vi "_CSMObj-Remove Internal Registry Rule.vi"(8 "Error In":errorcluster caption="Error in (no error)", 10 "Rule":string, 11 "CSMQ In":T1={"info"={"Module Name"="", "Requested Name"="", "Group Name"="", "Mode"=enum."Stand Alone", "Allowed Messages"=[]}, "Refs"={"WatchDogQ"=refnum, "CSMDataDVR"=refnum, "Queue"={"HPriorityQ"=refnum, "LowPriorityQ"=refnum}, "GroupDataDVR"=refnum, "TagMap"=refnum, "ExitEvent"=refnum, "NewStateEvent"=refnum, "StatusEvent"=refnum, "InterruptEvent"=refnum}}) -> (0 "Error Out":errorcluster, 3 "CSMQ Out":T1={"info"={"Module Name"="", "Requested Name"="", "Group Name"="", "Mode"=enum."Stand Alone", "Allowed Messages"=[]}, "Refs"={"WatchDogQ"=refnum, "CSMDataDVR"=refnum, "Queue"={"HPriorityQ"=refnum, "LowPriorityQ"=refnum}, "GroupDataDVR"=refnum, "TagMap"=refnum, "ExitEvent"=refnum, "NewStateEvent"=refnum, "StatusEvent"=refnum, "InterruptEvent"=refnum}})   [LabVIEW 2017, in "Communicable State Machine.lvlib"]
uses:
  Communicable State Machine.lvlib
  _CSMObj.ctl
  _CSMObj-Info.ctl
  Typedef/_CSM_MODE.ctl
  _CSMObj-Refs.ctl
  _CSMObj-Data.ctl
  Priority Queue/Priority Queue.ctl
  Typedef/_Cross CSM State Data.ctl
  Typedef/_CSM_MSG_TYPE.ctl
  Typedef/_Cross CSM State Response.ctl
  Typedef/_CSM_Response Source Message.ctl
  Priority Queue/def-Data(LowPRI-Q).ctl
  _CSMObj-ModeData.ctl
  Typedef/_CSM Status Change Event Data.ctl
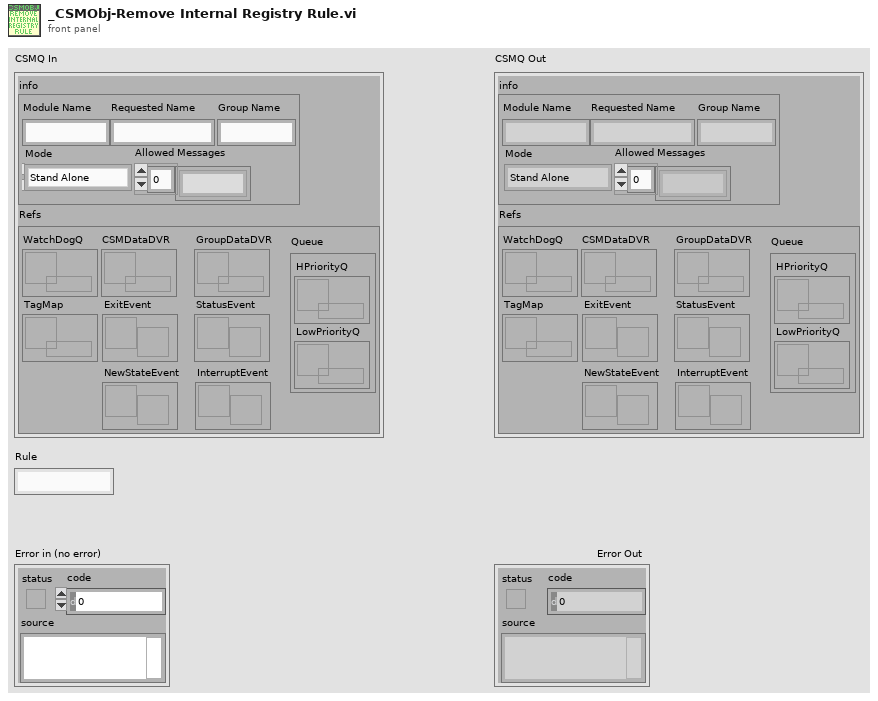
[diagram p1: front panel]
types:
  T1 = typedef "Communicable State Machine.lvlib/_CSMObj.ctl" = cluster{"info":T2, "Refs":T4}
  T2 = typedef "Communicable State Machine.lvlib/_CSMObj-Info.ctl" = cluster{"Module Name":string, "Requested Name":string, "Group Name":string, "Mode":T3, "Allowed Messages":string[]}
  T3 = typedef "Communicable State Machine.lvlib/_CSM_MODE.ctl" = enum16{"Not Exist", "Stand Alone", "CSM", "Worker", "Worker Agent", "Chain Node", "Chain"}
  T4 = typedef "Communicable State Machine.lvlib/_CSMObj-Refs.ctl" = cluster{"WatchDogQ":refnum<queue>, "CSMDataDVR":refnum<data-value>, "Queue":T5, "GroupDataDVR":refnum<data-value>, "TagMap":refnum<data-value>, "ExitEvent":refnum<user-event>, "NewStateEvent":refnum<user-event>, "StatusEvent":refnum<user-event>, "InterruptEvent":refnum<user-event>}
  T5 = typedef "Communicable State Machine.lvlib/Priority Queue.ctl" = cluster{"HPriorityQ":refnum<queue>, "LowPriorityQ":refnum<queue>}
  T6 = typedef "Communicable State Machine.lvlib/_CSMObj-Data.ctl" = cluster{"RemoteMessge?":bool, "error":errorcluster, "Return State":string, "Initialized":enum16{"Initializing", "Ready", "Exiting"}, "InternalRegistryRules":string[]}
  T7 = typedef "Communicable State Machine.lvlib/_CSMObj-ModeData.ctl" = cluster{"CSMDataDVR":refnum<data-value>[], "PriorityQueues":T5[], "Messages of Chain Nodes":cluster{"Module Name":string, "Allowed Messages":string[]}[], "Chain Message Mapping Map":variant, "SharedRegistryRules":string[]}
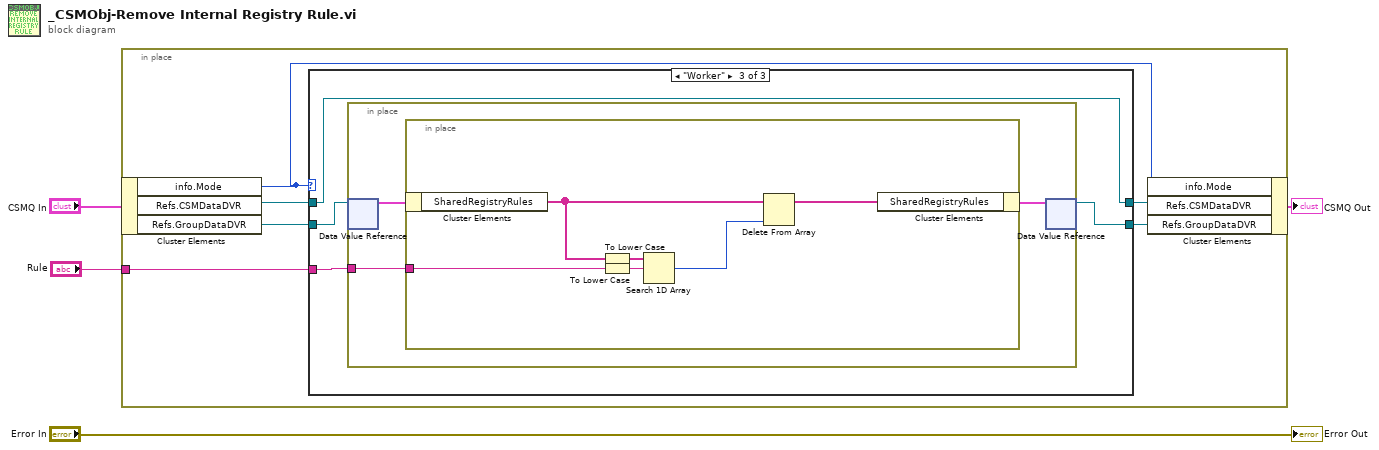
[diagram p0: block diagram]
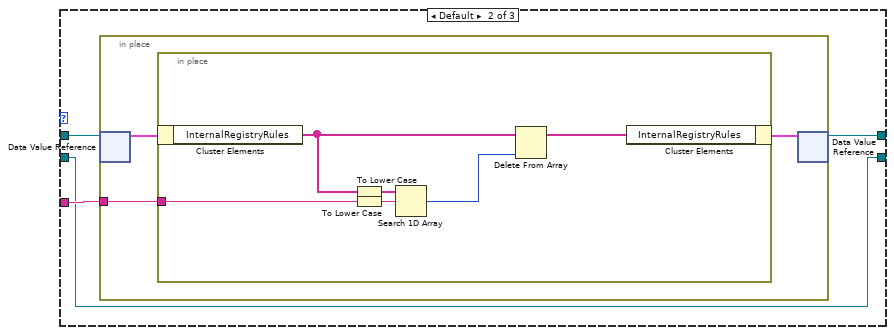
[diagram p3: hidden frame]
diagram:
  n1 = in-place "In Place Element Structure" {
    in-place-border: "Rule" -> [w8]
    n2 = in-place-cluster #1("CSMQ In") -> ("info.Mode"=w7:T3, "Refs.CSMDataDVR"=w10:refnum<data-value>, "Refs.GroupDataDVR"=w6:refnum<data-value>)
    n3 = case shown="\"Worker\"" w7 {
      tunnel: w10 -> [w12 w16 w26]
      tunnel: [w12 w15 w26] -> w9
      tunnel: w8 -> [_ w14 w29]
      tunnel: w6 -> [w11 w13 w28]
      tunnel: [w11 w13 w27] -> w5
      frame "Not Exist" {
      }
      frame Default {
        n4 = in-place {
          in-place-border: w14 -> [w17]
          n5 = in-place-dvr #2(w16) -> (w19:T6)  [unwired: 1 out]
          n6 = in-place {
            in-place-border: w17 -> [w23]
            n7 = in-place-cluster #3(w19) -> ("InternalRegistryRules"=w21:string[])
            n8 = To Lower Case(string=w21) -> (all lower case string=w25:string[])
            n9 = To Lower Case(string=w23) -> (all lower case string=w24:string)
            n10 = Search 1D Array(1D array=w25, element=w24) -> (index of element=w20:i32)  [unwired: 1 in]
            n11 = Delete From Array(array=w21, index=w20) -> (array with subset deleted=w22:string[])  [unwired: 1 in, 1 out]
            n12 = in-place-cluster #3("InternalRegistryRules"=w22) -> (w18:T6)
          }
          n13 = in-place-dvr #2(w18) -> (w15:refnum<data-value>)  [unwired: 1 out]
        }
      }
      frame "Worker" {
        n14 = in-place {
          in-place-border: w29 -> [w30]
          n15 = in-place-dvr #4(w28) -> (w32:T7)  [unwired: 1 out]
          n16 = in-place {
            in-place-border: w30 -> [w36]
            n17 = in-place-cluster #5(w32) -> ("SharedRegistryRules"=w34:string[])
            n18 = To Lower Case(string=w34) -> (all lower case string=w38:string[])
            n19 = To Lower Case(string=w36) -> (all lower case string=w37:string)
            n20 = Search 1D Array(1D array=w38, element=w37) -> (index of element=w33:i32)  [unwired: 1 in]
            n21 = Delete From Array(array=w34, index=w33) -> (array with subset deleted=w35:string[])  [unwired: 1 in, 1 out]
            n22 = in-place-cluster #5("SharedRegistryRules"=w35) -> (w31:T7)
          }
          n23 = in-place-dvr #4(w31) -> (w27:refnum<data-value>)  [unwired: 1 out]
        }
      }
    }
    n24 = in-place-cluster #1("info.Mode"=w7, "Refs.CSMDataDVR"=w9, "Refs.GroupDataDVR"=w5) -> (→"CSMQ Out":T1)
  }
  "Error Out" <- "Error In"
